vi "Sample_example.vi"() -> ()   [LabVIEW 2018]
uses:
  Sensor.lvclass
panel:
  out "data":T1
  out "Boolean":bool
  in  "stop":bool
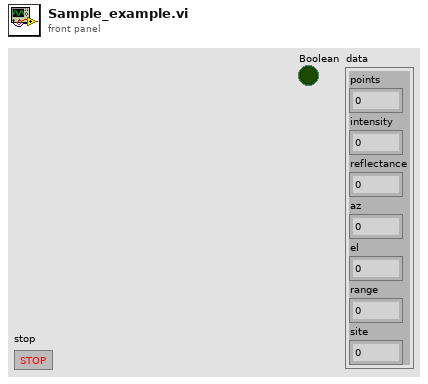
[diagram p1: front panel]
types:
  T1 = cluster{"points":u64, "intensity":u16, "reflectance":dbl, "az":dbl, "el":dbl, "range":dbl, "site":u8}
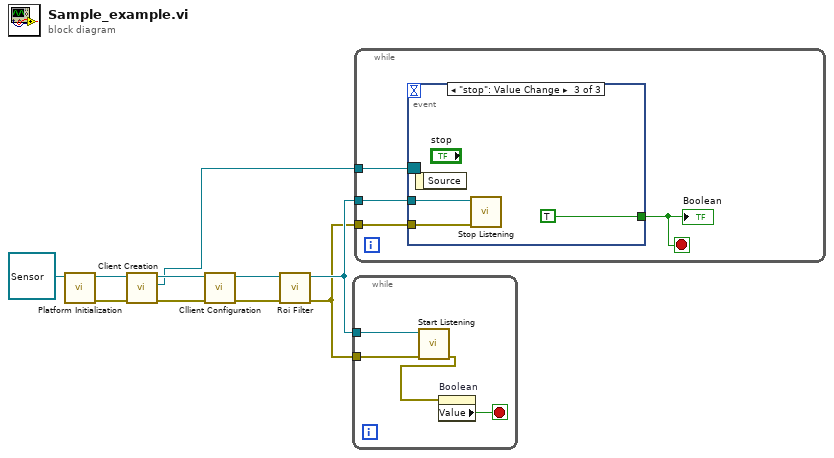
[diagram p0: block diagram]
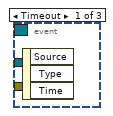
[diagram p2: hidden frame]
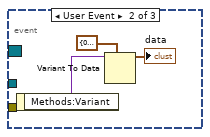
[diagram p3: hidden frame]
diagram:
  n1 = call-dynamic "Platform Initialization.vi"("Sensor in"=refnum<class "Sensor.lvclass"> refnum) -> ("error out"=w9:errorcluster, "Sensor out"=w10:refnum<class "Sensor.lvclass">)  [unwired: 9 in]
  n2 = call-dynamic "Client Creation.vi"("error in (no error)"=w9, "Sensor in"=w10) -> ("error out"=w8:errorcluster, "Event Registration Refnum"=w4:refnum<event-registration>, "Sensor out"=w7:refnum<class "Sensor.lvclass">)  [unwired: 7 in]
  n3 = call-dynamic "Cllient Configuration.vi"("error in (no error)"=w8, "Sensor in"=w7) -> ("error out"=w5:errorcluster, "Sensor out"=w6:refnum<class "Sensor.lvclass">)  [unwired: 8 in]
  n4 = call-dynamic "Roi Filter.vi"("error in (no error)"=w5, "Sensor in"=w6) -> ("error out"=w2:errorcluster, "Sensor out"=w3:refnum<class "Sensor.lvclass">)  [unwired: 8 in]
  n5 = while {
    tunnel: w3 -> [w14]
    tunnel: w2 -> [w11]
    stop <- w12 stop-if-true
    n6 = call-dynamic "Start Listening.vi"("error in (no error)"=w11, "Sensor in"=w14) -> ("error out"=w13:errorcluster)  [unwired: 8 in, 1 out]
    n7 = property on="Boolean" class="Bool (strict)"(error in=w13) -> ("Value"=w12:bool)  [unwired: 1 in, 2 out]
  }
  n8 = while {
    tunnel: w4 -> [w18]
    tunnel: w3 -> [w16]
    tunnel: w2 -> [w15]
    stop <- w17 stop-if-true
    n9 = event shown="[2] \"stop\": Value Change" {
      selector: w18 -> [_ _ _]
      dyn-events: _ -> [_ _ _]
      timeout: _ -> [_ _ _]
      tunnel: [_ _ TRUE] -> w17
      tunnel: w16 -> [_ _ w23]
      tunnel: w15 -> [_ _ w22]
      event Timeout {
        n10 = event-data() -> ()  [unwired: 1 in, 3 out]
      }
      event User Event {
        n11 = event-data() -> ("Methods:Variant"=w21:variant)  [unwired: 1 in]
        n12 = Variant To Data(type=T1 {"points"=0, "intensity"=0, "reflectance"=0.0, "az"=0.0, "el"=0.0, "range"=0.0, "site"=0} ("test"), Variant=w21) -> (data=→"data":T1)  [unwired: 1 in, 1 out]
      }
      event "stop": Value Change {
        n13 = event-data() -> ()  [unwired: 1 in, 1 out]
        n14 = call-dynamic "Stop Listening.vi"("error in (no error)"=w22, "Sensor in"=w23) -> ()  [unwired: 8 in, 2 out]
      }
    }
    "Boolean" <- w17
  }
